vi "New Knock Cylinder Cluster Constant.vi"(11 "Bitfile name":string) -> (3 "Knock":T1)   [LabVIEW 2013, in "Engine Simulation Toolkit System Explorer.lvlib"]
uses:
  Engine Simulation Toolkit System Explorer.lvlib
  Knock Cylinder.ctl
  Shared/Constants and GUIDs.vi
  Shared/Engine Simulation Toolkit Shared.lvlib
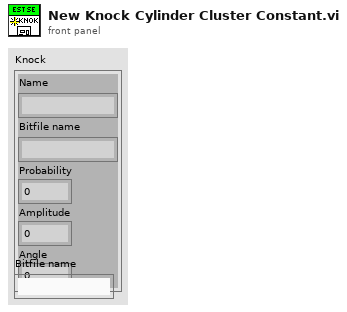
[diagram p1: front panel]
types:
  T1 = typedef "Engine Simulation Toolkit System Explorer.lvlib/Knock Cylinder.ctl" = cluster{"Name":string, "Bitfile name":string, "Probability":dbl, "Amplitude":dbl, "Angle":dbl}
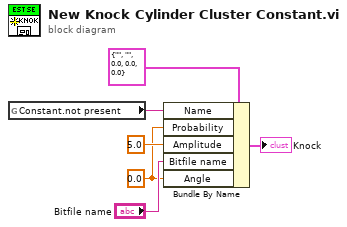
[diagram p0: block diagram]
diagram:
  w1 = 0.0 ("Probability")
  n1 = global read "Constants and GUIDs.vi" "Constant.not present"() -> (w5:string)
  n2 = Bundle By Name(cluster=T1 {"Name"="", "Bitfile name"="", "Probability"=0.0, "Amplitude"=0.0, "Angle"=0.0} ("Window"), "Name"=w5, "Probability"=w1, "Amplitude"=5.0, "Bitfile name"="Bitfile name", "Angle"=w1) -> (→"Knock":T1)
